vi "HTML_Table_Data.vi"(8 "entrée d'erreur (pas d'erreur)":errorcluster, 10 "Tableau":string[][](array[string]), 11 "chaîne en entrée":string) -> (0 "sortie d'erreur":errorcluster, 3 "result string":string)   [LabVIEW 2017]
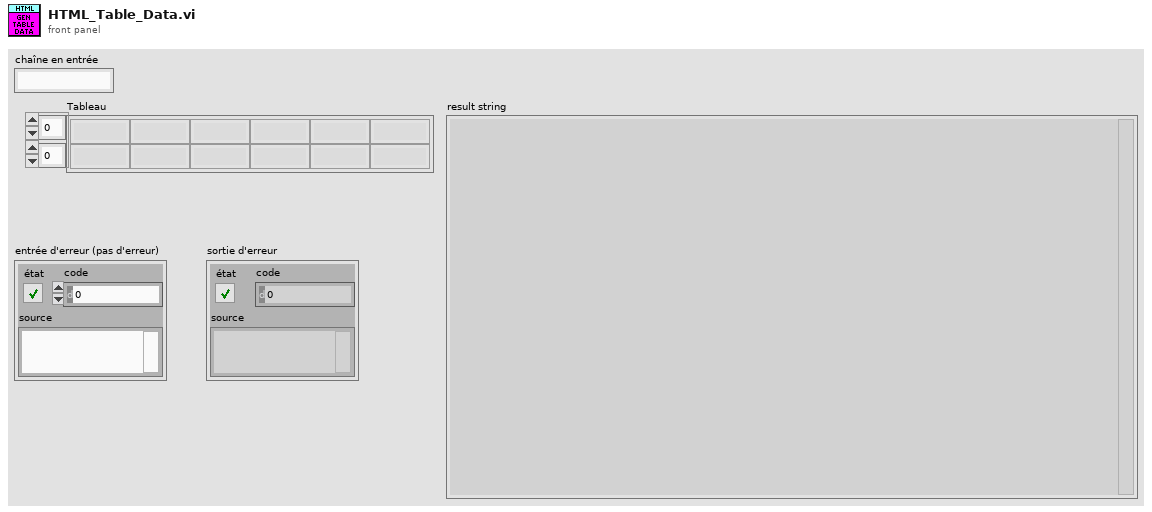
[diagram p1: front panel]
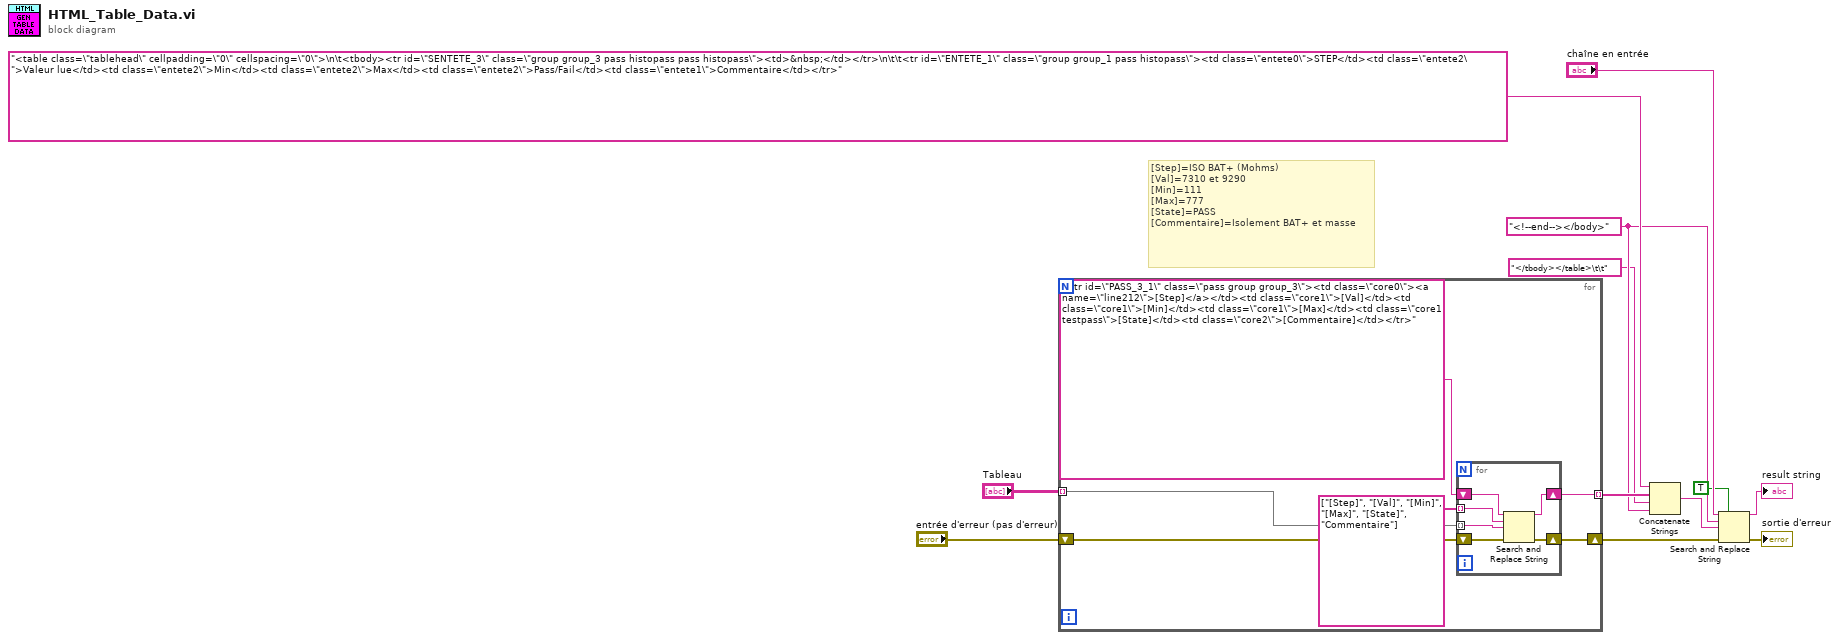
[diagram p0: block diagram]
diagram:
  w4 = "<!--end--></body>" ("chaîne recherchée")
  # "[Step]=ISO BAT+ (Mohms)\n[Val]=7310 et 9290\n[Min]=111\n[Max]=777\n[State]=PASS\n[Commentaire]=Isolement BAT+ et masse"
  n1 = for {
    tunnel: [w13] -> w9 mode=indexing
    shift-right: [w18] -> w10
    shift-left: "entrée d'erreur (pas d'erreur)" -> [w17]
    tunnel: "Tableau" -> [w15] mode=indexing
    n2 = for {
      tunnel: string[] ["[Step]", "[Val]", "[Min]", "[Max]", "[State]", "Commentaire"] -> [w24] mode=indexing
      tunnel: w15 -> [w23] mode=indexing
      shift-right: [w21] -> w18
      shift-left: w17 -> [w22]
      shift-right: [w19] -> w13
      shift-left: "<tr id=\"PASS_3_1\" class=\"pass group group_3\"><td class=\"core0\"><a name=\"line212\">[Step]</a></td><td class=\"core1\">[Val]</td><td class=\"core1\">[Min]</td><td class=\"core1\">[Max]</td><td class=\"core1 testpass\">[State]</td><td class=\"core2\">[Commentaire]</td></tr>" -> [w20]
      n3 = Search and Replace String(input string=w20, search string=w24, replace string=w23, error in=w22) -> (result string=w19:string, error out=w21:errorcluster)  [unwired: 4 in, 2 out]
    }
  }
  n4 = Concatenate Strings("<table class=\"tablehead\" cellpadding=\"0\" cellspacing=\"0\">\n\t<tbody><tr id=\"SENTETE_3\" class=\"group group_3 pass histopass pass histopass\"><td>&nbsp;</td></tr>\n\t\t<tr id=\"ENTETE_1\" class=\"group group_1 pass histopass\"><td class=\"entete0\">STEP</td><td class=\"entete2\">Valeur lue</td><td class=\"entete2\">Min</td><td class=\"entete2\">Max</td><td class=\"entete2\">Pass/Fail</td><td class=\"entete1\">Commentaire</td></tr>", w9, "</tbody></table>\t\t", w4) -> (w8:string)
  n5 = Search and Replace String(replace all?=TRUE ("tout remplacer ? (F)"), input string="chaîne en entrée", search string=w4, replace string=w8, error in=w10) -> (result string=→"result string":string, error out=→"sortie d'erreur":errorcluster)  [unwired: 3 in, 2 out]
